vi "Enable TSP Net Connection.vi"(0 "VISA resource name":refnum<visa-resource-name>, 1 "Remote ID Query (F: Disable)":bool, 2 "Termination (1: LF)":i32(ring)=1 items=["Nil", "LF", "CRLF", "LFCR", "CR"], 5 "Instrument ID":string, 7 "Enable Connection (T: Enable)":bool=TRUE, 9 "IP Address":string, 11 "error in (no error)":errorcluster, 12 "Port Number (5025)":i32=5025, 13 "Initialization String":string) -> (4 "VISA resource name out":refnum<visa-resource-name>, 15 "error out":errorcluster)   [LabVIEW 2019, in "Keithley 2600 Series.lvlib"]
doc: "Establishes a TSP net connection with another LAN interface."
uses:
  Keithley 2600 Series.lvlib
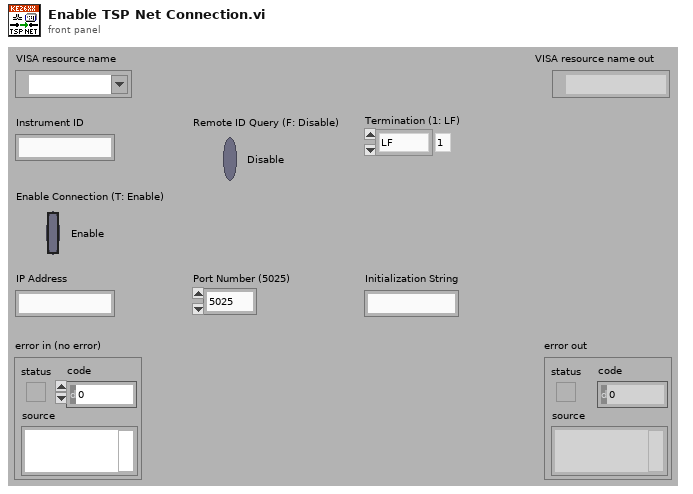
[diagram p1: front panel]
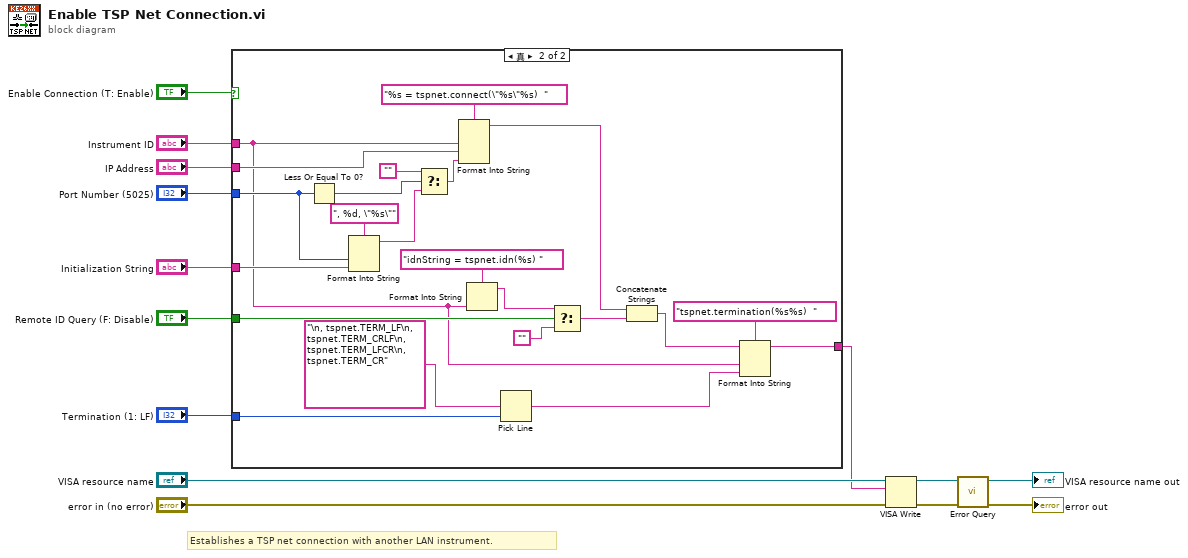
[diagram p0: block diagram]
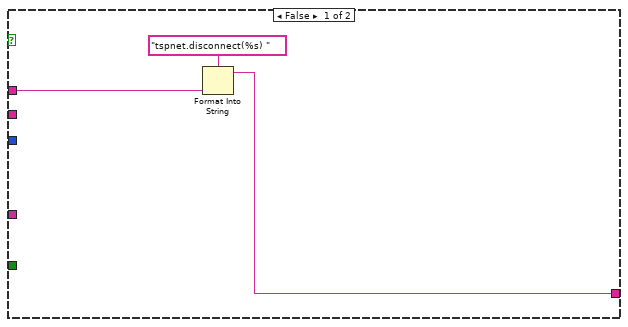
[diagram p2: hidden frame]
diagram:
  # "Establishes a TSP net connection with another LAN instrument."
  n1 = case shown="真" "Enable Connection (T: Enable)" {
    tunnel: "Instrument ID" -> [w16 w18]
    tunnel: "IP Address" -> [_ w38]
    tunnel: "Port Number (5025)" -> [_ w33]
    tunnel: "Initialization String" -> [_ w32]
    tunnel: [w15 w20] -> w6
    tunnel: "Remote ID Query (F: Disable)" -> [_ w29]
    tunnel: "Termination (1: LF)" -> [_ w19]
    frame False {
      n2 = Format Into String(format string="tspnet.disconnect(%s) ", w16) -> (resulting string=w15:string)  [unwired: 2 in, 1 out]
    }
    frame True {
      n3 = Less Or Equal To 0?(x=w33) -> (x <= 0?=w37:bool)
      n4 = Format Into String(format string=", %d, \"%s\"", w33, w32) -> (resulting string=w31:string)  [unwired: 2 in, 1 out]
      n5 = Select(t="", s=w37, f=w31) -> (s? t:f=w35:string)
      n6 = Format Into String(format string="%s = tspnet.connect(\"%s\"%s)  ", w18, w38, w35) -> (resulting string=w25:string)  [unwired: 2 in, 1 out]
      n7 = Format Into String(format string="idnString = tspnet.idn(%s) ", w18) -> (resulting string=w27:string)  [unwired: 2 in, 1 out]
      n8 = Pick Line(multi-line string="\n, tspnet.TERM_LF\n, tspnet.TERM_CRLF\n, tspnet.TERM_LFCR\n, tspnet.TERM_CR", line index=w19) -> (output string=w23:string)  [unwired: 1 in]
      n9 = Select(t=w27, s=w29, f="") -> (s? t:f=w26:string)
      n10 = Concatenate Strings(w25, w26) -> (w21:string)
      n11 = Format Into String(format string="tspnet.termination(%s%s)  ", initial string=w21, w18, w23) -> (resulting string=w20:string)  [unwired: 1 in, 1 out]
    }
  }
  n12 = VISA Write(VISA resource name="VISA resource name", write buffer=w6, error in (no error)="error in (no error)") -> (VISA resource name out=w13:refnum<visa-resource-name>, error out=w3:errorcluster)  [unwired: 1 out]
  n13 = call "Error Query.vi"("error in (no error)"=w3, "VISA resource name"=w13) -> ("error out"=→"error out":errorcluster, "VISA resource name out"=→"VISA resource name out":refnum<visa-resource-name>)  [unwired: 6 in, 2 out]
